vi "get_data.vi"(8 "error in (no error)":errorcluster, 11 "DoublyNodeRef in":refnum<class "DoublyNodeRef.lvclass">) -> (0 "error out":errorcluster, 2 "data":dbl, 3 "DoublyNodeRef out":refnum<class "DoublyNodeRef.lvclass">)   [LabVIEW 2021, in "DoublyNodeRef.lvclass"]
uses:
  DoublyNodeRef.lvclass
  DoublyNodeRef.lvclass/DoublyNodeRef.ctl
  IDoublyNode/IDoublyNode.lvclass
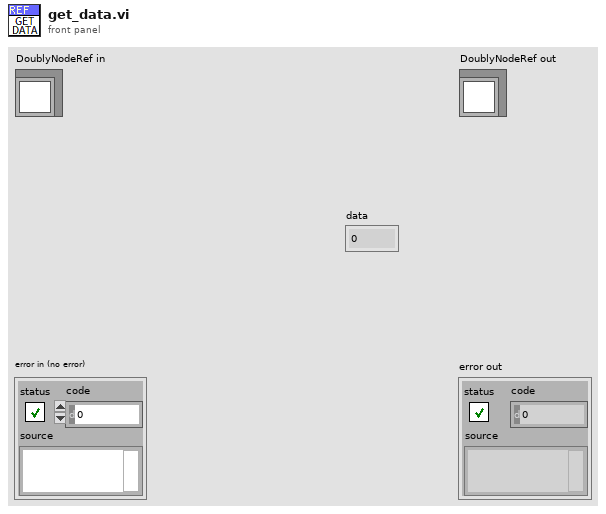
[diagram p1: front panel]
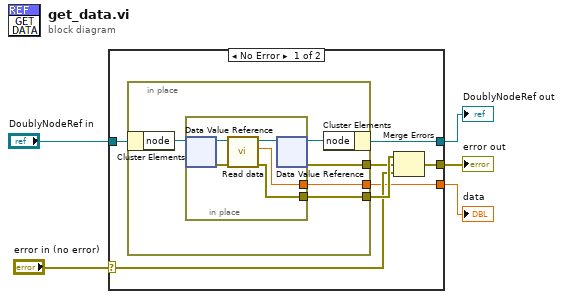
[diagram p0: block diagram]
diagram:
  n1 = case shown="No Error" "error in (no error)" {
    selector: "error in (no error)" -> [w9 w24]
    tunnel: [w8 w24] -> w1
    tunnel: "DoublyNodeRef in" -> [w12 w23]
    tunnel: [w7 _] -> w3
    tunnel: [w6 w23] -> w2
    frame No Error {
      n2 = in-place {
        in-place-border: [w15] -> w11
        in-place-border: [w14] -> w10
        in-place-border: [w13] -> w7
        n3 = in-place-cluster #1(w12) -> ("node"=w17:refnum<data-value>)
        n4 = in-place {
          in-place-border: [w19] -> w15
          in-place-border: [w18] -> w13
          n5 = in-place-dvr #2(w17) -> (w21:refnum<class "IDoublyNode.lvclass">, w22:errorcluster)
          n6 = call-dynamic "Read data.vi"("error in (no error)"=w22, "IDoublyNode in"=w21) -> ("error out"=w19:errorcluster, "data"=w18:dbl, "IDoublyNode out"=w20:refnum<class "IDoublyNode.lvclass">)  [unwired: 7 in]
          n7 = in-place-dvr #2(w20) -> (w16:refnum<data-value>, w14:errorcluster)
        }
        n8 = in-place-cluster #1("node"=w16) -> (w6:refnum<class "DoublyNodeRef.lvclass">)
      }
      n9 = Merge Errors(w11, w10, w9) -> (w8:errorcluster)
    }
    frame Error {
    }
  }
  "error out" <- w1
  "DoublyNodeRef out" <- w2
  "data" <- w3
